vi "COMMAND_ResetController.vi"(8 "error in (no error)":errorcluster, 11 "MH100301DMC in":refnum<class "StageMH100301DMC.lvclass">) -> (0 "error out":errorcluster, 3 "MH100301DMC out":refnum<class "StageMH100301DMC.lvclass">)   [LabVIEW 2010, in "StageMH100301DMC.lvclass"]
uses:
  StageMH100301DMC.lvclass
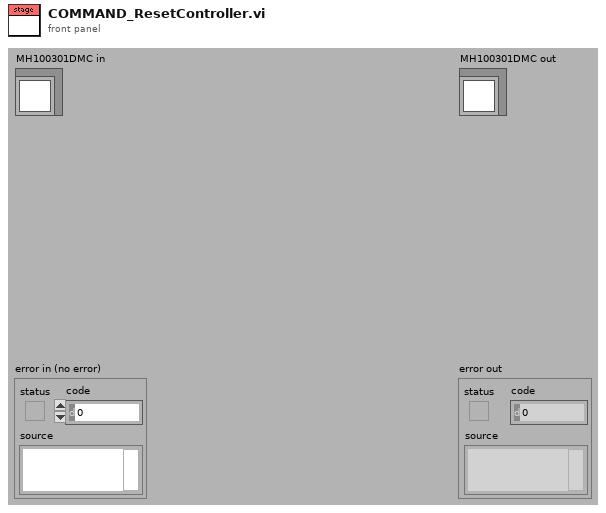
[diagram p1: front panel]
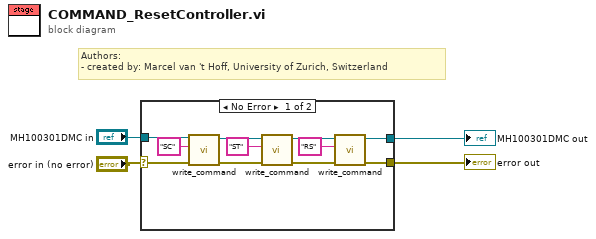
[diagram p0: block diagram]
diagram:
  # "Authors: \n- created by: Marcel van 't Hoff, University of Zurich, Switzerland"
  n1 = case shown="No Error" "error in (no error)" {
    selector: "error in (no error)" -> [w14 w17]
    tunnel: [w7 w17] -> w3
    tunnel: [w8 w16] -> w1
    tunnel: "MH100301DMC in" -> [w13 w16]
    frame No Error {
      n2 = call-dynamic "write_command.vi"("error in (no error)"=w14, "command (without terminating \"\\n\")"="SC" ("command (without terminating \"\\n\")"), "MH100301DMC in"=w13) -> ("error out"=w5:errorcluster, "MH100301DMC out"=w10:refnum<class "StageMH100301DMC.lvclass">)  [unwired: 6 in, 1 out]
      n3 = call-dynamic "write_command.vi"("error in (no error)"=w5, "command (without terminating \"\\n\")"="ST" ("command (without terminating \"\\n\")"), "MH100301DMC in"=w10) -> ("error out"=w6:errorcluster, "MH100301DMC out"=w9:refnum<class "StageMH100301DMC.lvclass">)  [unwired: 6 in, 1 out]
      n4 = call-dynamic "write_command.vi"("error in (no error)"=w6, "command (without terminating \"\\n\")"="RS" ("command (without terminating \"\\n\")"), "MH100301DMC in"=w9) -> ("error out"=w7:errorcluster, "MH100301DMC out"=w8:refnum<class "StageMH100301DMC.lvclass">)  [unwired: 6 in, 1 out]
    }
    frame Error {
    }
  }
  "error out" <- w3
  "MH100301DMC out" <- w1
